vi "add_line_to_enface_interp.vi"(0 "En Face Image":T1, 1 "Shift":dbl=1.0, 5 "Raw Image":T1, 7 "Add Height":dbl=1.0, 9 "Input Line":dbl=1.0, 11 "error in (no error)":errorcluster, 12 "Output Line":dbl) -> (4 "En Face Image Out":T1, 15 "error out":errorcluster)   [LabVIEW 2016]
doc: "Adds the next line to the en face or fluorescence image. The raw images can either be an OCT B-scan, in which case a single depth line (T scan) is extracted or a fluorescence line, in which case 'input line must be set to zero. If we have moved more then one line in the output image then the input line is simply copied multiple times to fill the space (zero order interpolation)"
uses:
  <vilib>/vision/Image Controls.llb/IMAQ Image.ctl
  <vilib>/vision/NI_Vision_Development_Module.lvlib
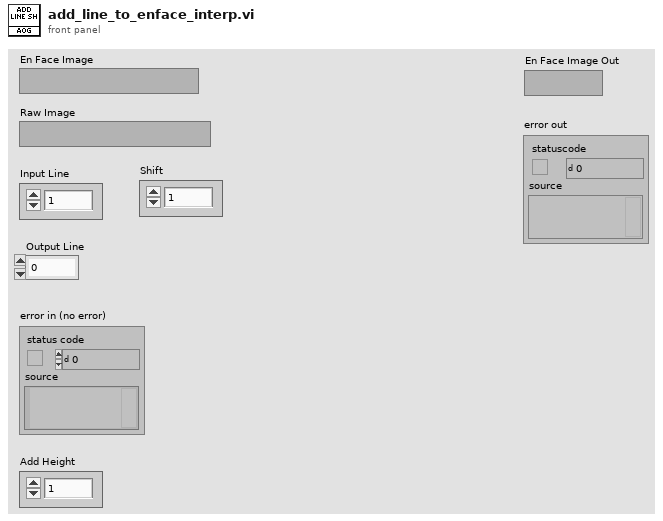
[diagram p1: front panel]
types:
  T1 = typedef "IMAQ Image.ctl" = refnum<image>
  T2 = typedef "Image Type" = u32
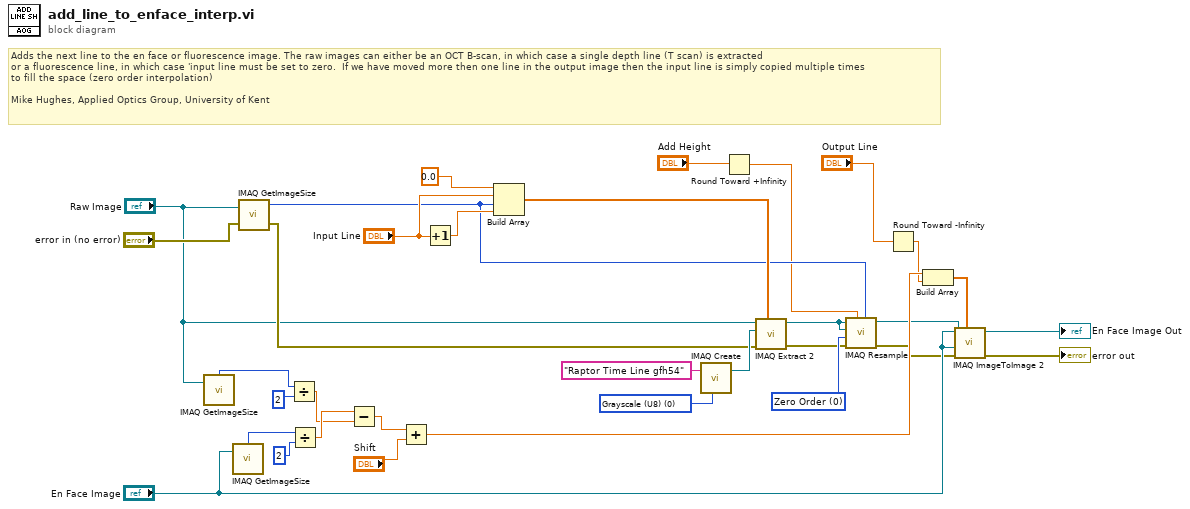
[diagram p0: block diagram]
diagram:
  w9 = u32 0 items=["Zero Order", "Bi-Linear", "Quadratic", "Cubic Spline"] ("Interpolation Type")
  w31 = T2 0 items=["Grayscale (U8)", "Grayscale (I16)", "Grayscale (SGL)", "Complex (CSG)", "RGB (U32)", "HSL (U32)", "RGB (U64)", "Grayscale (U16)"] ("Image Type")
  # "Adds the next line to the en face or fluorescence image. The raw images can either be an OCT B-scan, in which case a single depth line (T scan) is extracted\nor a fluorescence line, in which case 'input line must be set to zero.  If we have moved more then one line in the output image then the input line is simply copied multiple times\nto fill the space (zero order interpolation)\n\nMike Hughes, Applied Optics Group, University of Kent"
  n1 = call "IMAQ GetImageSize"("Image"="Raw Image") -> ("X Resolution"=w16:i32)  [unwired: 3 in, 2 out]
  n2 = call "IMAQ GetImageSize"("Image"="En Face Image") -> ("X Resolution"=w20:i32)  [unwired: 3 in, 2 out]
  n3 = call "IMAQ GetImageSize"("Image"="Raw Image", "error in (no error)"="error in (no error)") -> ("X Resolution"=w8:i32, "error out"=w24:errorcluster)  [unwired: 2 in, 1 out]
  n4 = Divide(x=w16, y=2) -> (x/y=w14:dbl)
  n5 = Divide(x=w20, y=2) -> (x/y=w15:dbl)
  n6 = Subtract(x=w15, y=w14) -> (x-y=w13:dbl)
  n7 = Add(x=w13, y="Shift") -> (x+y=w11:dbl)
  n8 = Increment(x="Input Line") -> (x+1=w22:dbl)
  n9 = Build Array(0.0 ("element"), "Input Line", w8, w22) -> (w29:dbl[])
  n10 = call "IMAQ Create"("Image Name"="Raptor Time Line gfh54", "Image Type"=w31) -> ("New Image"=w30:T1)  [unwired: 3 in, 1 out]
  n11 = Round Toward +Infinity(x="Add Height") -> (ceil(x): smallest int >= x=w1:dbl)
  n12 = call "IMAQ Extract 2"("Optional Rectangle"=w29, "error in (no error)"=w24, "Image Dst"=w30, "Image Src"="Raw Image") -> ("error out"=w5:errorcluster, "Image Dst Out"=w10:T1)  [unwired: 6 in]
  n13 = call "IMAQ Resample"("X Resolution"=w8, "Y Resolution"=w1, "error in (no error)"=w5, "Interpolation Type"=w9, "Image Dst"=w10, "Image Src"=w10) -> ("error out"=w6:errorcluster, "Image Dst Out"=w7:T1)  [unwired: 4 in]
  n14 = Round Toward -Infinity(1:"Output Line") -> (0:w4:dbl)
  n15 = Build Array(w11, w4) -> (w28:dbl[])
  n16 = call "IMAQ ImageToImage 2"("Offset Left/Top"=w28, "error in (no error)"=w6, "Image Dst"="En Face Image", "Image Src (Small)"=w7, "Image Src (Large)"="En Face Image") -> ("error out"=→"error out":errorcluster, "Image Dst Out"=→"En Face Image Out":T1)  [unwired: 5 in]
